vi "DACSetBoardRange.vi"(7 "DeviceIndex":u32, 8 "error in (no error)":errorcluster) -> (0 "error out":errorcluster)   [LabVIEW 2011]
doc: "unsigned long CTR_8254SelectGate( - This function selects a counter for use as the gate in\nfrequency measurement on other counters, and starts the .\nunsigned long DeviceIndex - number from 0-31 indicating which device you wish to select a gate\nfor\nunsigned long GateIndex - number from 0-14 indicating which counter you wish to select as a\ngate; this is in \"blockless\" addressing\n)\nThis function is currently only supported by the USB-CTR-15."
uses:
  AIOUSB.dll
panel:
  in  "Range Code":u32
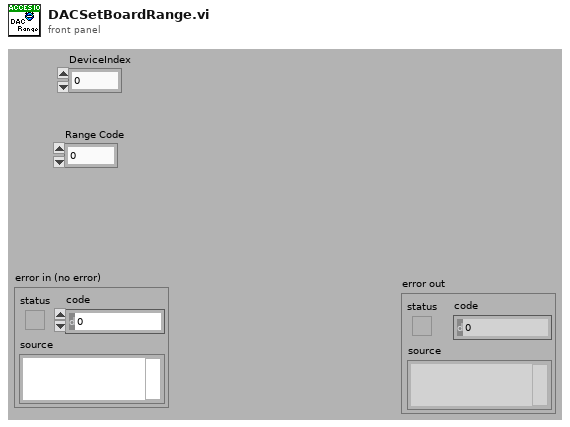
[diagram p1: front panel]
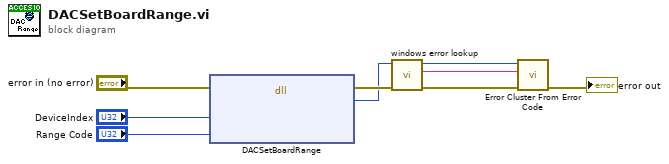
[diagram p0: block diagram]
diagram:
  n1 = dll-call lib="AIOUSB.dll" fn="DACSetBoardRange"(error in="error in (no error)", "DeviceIndex"="DeviceIndex", "RangeCode"="Range Code") -> (error out=w5:errorcluster, "return type"=w4:u32)  [unwired: 4 in, 1 out]
  n2 = call <instrlib>:"windows error lookup.vi"("error in (no error)"=w5, "Error Code"=w4) -> ("error out"=w7:errorcluster, "error message (\"\")"=w8:string)  [unwired: 8 in]
  n3 = call <vilib>:"Error Cluster From Error Code.vi"("error in (no error)"=w7, "error message (\"\")"=w8, "error code (0)"=w4) -> ("error out"=→"error out":errorcluster)  [unwired: 6 in]
